vi "setUp.vi"(8 "error in (no error)":errorcluster, 11 "reference in":refnum<class "Configuration Tests.lvclass">) -> (0 "error out":errorcluster, 3 "reference out":refnum<class "Configuration Tests.lvclass">)   [LabVIEW 2017, in "Configuration Tests.lvclass"]
doc: "setUp runs prior to the test method during test execution. Use this method to initialize any object data required by your tests."
uses:
  Configuration Tests.lvclass
  C:/Program Files (x86)/National Instruments/LabVIEW 2017/vi.lib/addons/_JKI Toolkits/VI Tester/TestCase.llb/TestCase.lvclass
  Typedefs/DSF Engine Framework Configuration.ctl
  Typedefs/DSF Engine Plugin Configuration.ctl
  Typedefs/DSF Timing Info.ctl
  Typedefs/DSF Engine Plugin Thread Configuration.ctl
  Typedefs/DSF Settings Info.ctl
  Typedefs/DSF Engine Transfer Group Configuration.ctl
  Typedefs/DSF Direction.ctl
  Typedefs/DSF Engine Transfer Configuration.ctl
  Typedefs/DSF Byte Order.ctl
  Typedefs/DSF Engine Channel Configuration.ctl
  Typedefs/DSF Data Type.ctl
  Typedefs/DSF Timeout Behavior.ctl
  Configuration Tests.lvclass/Configuration Tests.ctl
  <vilib>/addons/_JKI Toolkits/VI Tester/TestCase.llb/TestCase.lvclass
  DSF Core.lvlib
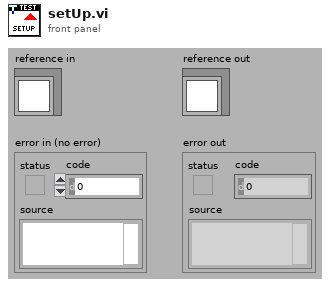
[diagram p1: front panel]
types:
  T1 = typedef "DSF Core.lvlib/DSF Engine Framework Configuration.ctl" = cluster{"plugins":T2[]}
  T2 = typedef "DSF Core.lvlib/DSF Engine Plugin Configuration.ctl" = cluster{"name":string, "components":string[], "cycle timing":T3, "threads":T4[], "transfer groups":T6[], "settings":T5}
  T3 = typedef "DSF Core.lvlib/DSF Timing Info.ctl" = cluster{"priority":u64, "decimation":u64, "offset":u64}
  T4 = typedef "DSF Core.lvlib/DSF Engine Plugin Thread Configuration.ctl" = cluster{"processor":i32, "priority offset":i16, "settings":T5}
  T5 = typedef "DSF Core.lvlib/DSF Settings Info.ctl" = cluster{"component":string, "name":string, "values":cluster{"key":string, "value":string}[]}[]
  T6 = typedef "DSF Core.lvlib/DSF Engine Transfer Group Configuration.ctl" = cluster{"name":string, "direction":T7, "cycle timing":T3, "thread index":u8, "settings":T5, "transfers":T8[], "timeout behavior":T12, "convert buffers":bool}
  T7 = typedef "DSF Core.lvlib/DSF Direction.ctl" = enum8{"Tx", "Rx"}
  T8 = typedef "DSF Core.lvlib/DSF Engine Transfer Configuration.ctl" = cluster{"name":string, "string byte order":T9, "settings":T5, "channels":T10[]}
  T9 = typedef "DSF Core.lvlib/DSF Byte Order.ctl" = enum8{"big-endian", "little-endian"}
  T10 = typedef "DSF Core.lvlib/DSF Engine Channel Configuration.ctl" = cluster{"string offset":u64, "name":string, "units":string, "engine data type":T11, "string data type":T11, "settings":T5}
  T11 = typedef "DSF Core.lvlib/DSF Data Type.ctl" = enum8{"Bool", "SGL", "DBL", "I8", "I16", "I32", "I64", "U8", "U16", "U32", "U64"}
  T12 = typedef "DSF Core.lvlib/DSF Timeout Behavior.ctl" = enum8{"Increment Late Count", "Throw Error"}
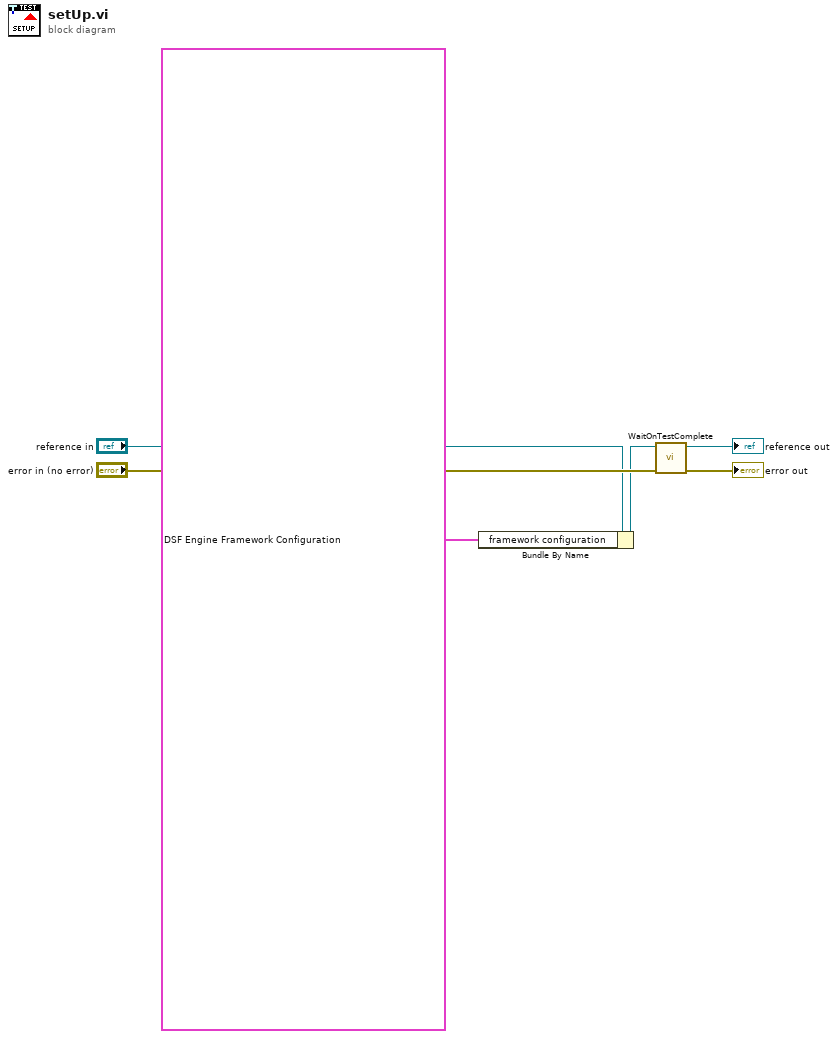
[diagram p0: block diagram]
diagram:
  n1 = Bundle By Name(cluster="reference in", "framework configuration"=T1 {"plugins"=[{"name"="Plugin", "components"=[], "cycle timing"={"priority"=10000, "decimation"=1, "offset"=0}, "threads"=[{"processor"=-2, "priority offset"=0, "settings"=[{"component"="a", "name"="a", "values"=[{"key"="a", "value"="a"}]}]}], "transfer groups"=[{"name"="Group", "direction"=enum."Tx", "cycle timing"={"priority"=100, "decimation"=1, "offset"=0}, "thread index"=255, "settings"=[{"component"="a", "name"="a", "values"=[{"key"="a", "value"="a"}]}], "transfers"=[{"name"="Transfer", "string byte order"=enum."big-endian", "settings"=[{"component"="a", "name"="a", "values"=[{"key"="a", "value"="a"}]}], "channels"=[{"string offset"=0, "name"="Channel", "units"="V", "engine data type"=enum."DBL", "string data type"=enum."DBL", "settings"=[]}, {"string offset"=0, "name"="Channel", "units"="V", "engine data type"=enum."DBL", "string data type"=enum."DBL", "settings"=[]}, {"string offset"=0, "name"="Channel", "units"="V", "engine data type"=enum."DBL", "string data type"=enum."DBL", "settings"=[]}, {"string offset"=0, "name"="Channel", "units"="V", "engine data type"=enum."DBL", "string data type"=enum."DBL", "settings"=[]}, {"string offset"=0, "name"="Channel", "units"="V", "engine data type"=enum."DBL", "string data type"=enum."DBL", "settings"=[]}, {"string offset"=0, "name"="Channel", "units"="V", "engine data type"=enum."DBL", "string data type"=enum."DBL", "settings"=[]}, {"string offset"=0, "name"="Channel", "units"="V", "engine data type"=enum."DBL", "string data type"=enum."DBL", "settings"=[]}, {"string offset"=0, "name"="Channel", "units"="V", "engine data type"=enum."DBL", "string data type"=enum."DBL", "settings"=[]}, {"string offset"=0, "name"="Channel", "units"="V", "engine data type"=enum."DBL", "string data type"=enum."DBL", "settings"=[]}, {"string offset"=0, "name"="Channel", "units"="V", "engine data type"=enum."DBL", "string data type"=enum."DBL", "settings"=[]}, {"string offset"=0, "name"="Channel", "units"="V", "engine data type"=enum."DBL", "string data type"=enum."DBL", "settings"=[]}, {"string offset"=0, "name"="Channel", "units"="V", "engine data type"=enum."DBL", "string data type"=enum."DBL", "settings"=[]}, {"string offset"=0, "name"="Channel", "units"="V", "engine data type"=enum."DBL", "string data type"=enum."DBL", "settings"=[]}, {"string offset"=0, "name"="Channel", "units"="V", "engine data type"=enum."DBL", "string data type"=enum."DBL", "settings"=[]}, {"string offset"=0, "name"="Channel", "units"="V", "engine data type"=enum."DBL", "string data type"=enum."DBL", "settings"=[]}, {"string offset"=0, "name"="Channel", "units"="V", "engine data type"=enum."DBL", "string data type"=enum."DBL", "settings"=[]}, {"string offset"=0, "name"="Channel", "units"="V", "engine data type"=enum."DBL", "string data type"=enum."DBL", "settings"=[]}, {"string offset"=0, "name"="Channel", "units"="V", "engine data type"=enum."DBL", "string data type"=enum."DBL", "settings"=[]}, {"string offset"=0, "name"="Channel", "units"="V", "engine data type"=enum."DBL", "string data type"=enum."DBL", "settings"=[]}, {"string offset"=0, "name"="Channel", "units"="V", "engine data type"=enum."DBL", "string data type"=enum."DBL", "settings"=[]}, {"string offset"=0, "name"="Channel", "units"="V", "engine data type"=enum."DBL", "string data type"=enum."DBL", "settings"=[]}, {"string offset"=0, "name"="Channel", "units"="V", "engine data type"=enum."DBL", "string data type"=enum."DBL", "settings"=[]}, {"string offset"=0, "name"="Channel", "units"="V", "engine data type"=enum."DBL", "string data type"=enum."DBL", "settings"=[]}, {"string offset"=0, "name"="Channel", "units"="V", "engine data type"=enum."DBL", "string data type"=enum."DBL", "settings"=[]}, {"string offset"=0, "name"="Channel", "units"="V", "engine data type"=enum."DBL", "string data type"=enum."DBL", "settings"=[]}, {"string offset"=0, "name"="Channel", "units"="V", "engine data type"=enum."DBL", "string data type"=enum."DBL", "settings"=[]}, {"string offset"=0, "name"="Channel", "units"="V", "engine data type"=enum."DBL", "string data type"=enum."DBL", "settings"=[]}, {"string offset"=0, "name"="Channel", "units"="V", "engine data type"=enum."DBL", "string data type"=enum."DBL", "settings"=[]}, {"string offset"=0, "name"="Channel", "units"="V", "engine data type"=enum."DBL", "string data type"=enum."DBL", "settings"=[]}, {"string offset"=0, "name"="Channel", "units"="V", "engine data type"=enum."DBL", "string data type"=enum."DBL", "settings"=[]}, {"string offset"=0, "name"="Channel", "units"="V", "engine data type"=enum."DBL", "string data type"=enum."DBL", "settings"=[]}, {"string offset"=0, "name"="Channel", "units"="V", "engine data type"=enum."DBL", "string data type"=enum."DBL", "settings"=[]}, {"string offset"=0, "name"="Channel", "units"="V", "engine data type"=enum."DBL", "string data type"=enum."DBL", "settings"=[]}, {"string offset"=0, "name"="Channel", "units"="V", "engine data type"=enum."DBL", "string data type"=enum."DBL", "settings"=[]}, {"string offset"=0, "name"="Channel", "units"="V", "engine data type"=enum."DBL", "string data type"=enum."DBL", "settings"=[]}, {"string offset"=0, "name"="Channel", "units"="V", "engine data type"=enum."DBL", "string data type"=enum."DBL", "settings"=[]}, {"string offset"=0, "name"="Channel", "units"="V", "engine data type"=enum."DBL", "string data type"=enum."DBL", "settings"=[]}, {"string offset"=0, "name"="Channel", "units"="V", "engine data type"=enum."DBL", "string data type"=enum."DBL", "settings"=[]}, {"string offset"=0, "name"="Channel", "units"="V", "engine data type"=enum."DBL", "string data type"=enum."DBL", "settings"=[]}, {"string offset"=0, "name"="Channel", "units"="V", "engine data type"=enum."DBL", "string data type"=enum."DBL", "settings"=[]}, {"string offset"=0, "name"="Channel", "units"="V", "engine data type"=enum."DBL", "string data type"=enum."DBL", "settings"=[]}, {"string offset"=0, "name"="Channel", "units"="V", "engine data type"=enum."DBL", "string data type"=enum."DBL", "settings"=[]}, {"string offset"=0, "name"="Channel", "units"="V", "engine data type"=enum."DBL", "string data type"=enum."DBL", "settings"=[]}, {"string offset"=0, "name"="Channel", "units"="V", "engine data type"=enum."DBL", "string data type"=enum."DBL", "settings"=[]}, {"string offset"=0, "name"="Channel", "units"="V", "engine data type"=enum."DBL", "string data type"=enum."DBL", "settings"=[]}, {"string offset"=0, "name"="Channel", "units"="V", "engine data type"=enum."DBL", "string data type"=enum."DBL", "settings"=[]}, {"string offset"=0, "name"="Channel", "units"="V", "engine data type"=enum."DBL", "string data type"=enum."DBL", "settings"=[]}, {"string offset"=0, "name"="Channel", "units"="V", "engine data type"=enum."DBL", "string data type"=enum."DBL", "settings"=[]}, {"string offset"=0, "name"="Channel", "units"="V", "engine data type"=enum."DBL", "string data type"=enum."DBL", "settings"=[]}, {"string offset"=0, "name"="Channel", "units"="V", "engine data type"=enum."DBL", "string data type"=enum."DBL", "settings"=[]}, {"string offset"=0, "name"="Channel", "units"="V", "engine data type"=enum."DBL", "string data type"=enum."DBL", "settings"=[]}, {"string offset"=0, "name"="Channel", "units"="V", "engine data type"=enum."DBL", "string data type"=enum."DBL", "settings"=[]}, {"string offset"=0, "name"="Channel", "units"="V", "engine data type"=enum."DBL", "string data type"=enum."DBL", "settings"=[]}, {"string offset"=0, "name"="Channel", "units"="V", "engine data type"=enum."DBL", "string data type"=enum."DBL", "settings"=[]}, {"string offset"=0, "name"="Channel", "units"="V", "engine data type"=enum."DBL", "string data type"=enum."DBL", "settings"=[]}, {"string offset"=0, "name"="Channel", "units"="V", "engine data type"=enum."DBL", "string data type"=enum."DBL", "settings"=[]}, {"string offset"=0, "name"="Channel", "units"="V", "engine data type"=enum."DBL", "string data type"=enum."DBL", "settings"=[]}, {"string offset"=0, "name"="Channel", "units"="V", "engine data type"=enum."DBL", "string data type"=enum."DBL", "settings"=[]}, {"string offset"=0, "name"="Channel", "units"="V", "engine data type"=enum."DBL", "string data type"=enum."DBL", "settings"=[]}, {"string offset"=0, "name"="Channel", "units"="V", "engine data type"=enum."DBL", "string data type"=enum."DBL", "settings"=[]}, {"string offset"=0, "name"="Channel", "units"="V", "engine data type"=enum."DBL", "string data type"=enum."DBL", "settings"=[]}, {"string offset"=0, "name"="Channel", "units"="V", "engine data type"=enum."DBL", "string data type"=enum."DBL", "settings"=[]}, {"string offset"=0, "name"="Channel", "units"="V", "engine data type"=enum."DBL", "string data type"=enum."DBL", "settings"=[]}, {"string offset"=0, "name"="Channel", "units"="V", "engine data type"=enum."DBL", "string data type"=enum."DBL", "settings"=[]}, {"string offset"=0, "name"="Channel", "units"="V", "engine data type"=enum."DBL", "string data type"=enum."DBL", "settings"=[]}, {"string offset"=0, "name"="Channel", "units"="V", "engine data type"=enum."DBL", "string data type"=enum."DBL", "settings"=[]}, {"string offset"=0, "name"="Channel", "units"="V", "engine data type"=enum."DBL", "string data type"=enum."DBL", "settings"=[]}, {"string offset"=0, "name"="Channel", "units"="V", "engine data type"=enum."DBL", "string data type"=enum."DBL", "settings"=[]}, {"string offset"=0, "name"="Channel", "units"="V", "engine data type"=enum."DBL", "string data type"=enum."DBL", "settings"=[]}, {"string offset"=0, "name"="Channel", "units"="V", "engine data type"=enum."DBL", "string data type"=enum."DBL", "settings"=[]}, {"string offset"=0, "name"="Channel", "units"="V", "engine data type"=enum."DBL", "string data type"=enum."DBL", "settings"=[]}, {"string offset"=0, "name"="Channel", "units"="V", "engine data type"=enum."DBL", "string data type"=enum."DBL", "settings"=[]}, {"string offset"=0, "name"="Channel", "units"="V", "engine data type"=enum."DBL", "string data type"=enum."DBL", "settings"=[]}, {"string offset"=0, "name"="Channel", "units"="V", "engine data type"=enum."DBL", "string data type"=enum."DBL", "settings"=[]}, {"string offset"=0, "name"="Channel", "units"="V", "engine data type"=enum."DBL", "string data type"=enum."DBL", "settings"=[]}, {"string offset"=0, "name"="Channel", "units"="V", "engine data type"=enum."DBL", "string data type"=enum."DBL", "settings"=[]}, {"string offset"=0, "name"="Channel", "units"="V", "engine data type"=enum."DBL", "string data type"=enum."DBL", "settings"=[]}, {"string offset"=0, "name"="Channel", "units"="V", "engine data type"=enum."DBL", "string data type"=enum."DBL", "settings"=[]}, {"string offset"=0, "name"="Channel", "units"="V", "engine data type"=enum."DBL", "string data type"=enum."DBL", "settings"=[]}, {"string offset"=0, "name"="Channel", "units"="V", "engine data type"=enum."DBL", "string data type"=enum."DBL", "settings"=[]}, {"string offset"=0, "name"="Channel", "units"="V", "engine data type"=enum."DBL", "string data type"=enum."DBL", "settings"=[]}, {"string offset"=0, "name"="Channel", "units"="V", "engine data type"=enum."DBL", "string data type"=enum."DBL", "settings"=[]}, {"string offset"=0, "name"="Channel", "units"="V", "engine data type"=enum."DBL", "string data type"=enum."DBL", "settings"=[]}, {"string offset"=0, "name"="Channel", "units"="V", "engine data type"=enum."DBL", "string data type"=enum."DBL", "settings"=[]}, {"string offset"=0, "name"="Channel", "units"="V", "engine data type"=enum."DBL", "string data type"=enum."DBL", "settings"=[]}, {"string offset"=0, "name"="Channel", "units"="V", "engine data type"=enum."DBL", "string data type"=enum."DBL", "settings"=[]}, {"string offset"=0, "name"="Channel", "units"="V", "engine data type"=enum."DBL", "string data type"=enum."DBL", "settings"=[]}, {"string offset"=0, "name"="Channel", "units"="V", "engine data type"=enum."DBL", "string data type"=enum."DBL", "settings"=[]}, {"string offset"=0, "name"="Channel", "units"="V", "engine data type"=enum."DBL", "string data type"=enum."DBL", "settings"=[]}, {"string offset"=0, "name"="Channel", "units"="V", "engine data type"=enum."DBL", "string data type"=enum."DBL", "settings"=[]}, {"string offset"=0, "name"="Channel", "units"="V", "engine data type"=enum."DBL", "string data type"=enum."DBL", "settings"=[]}, {"string offset"=0, "name"="Channel", "units"="V", "engine data type"=enum."DBL", "string data type"=enum."DBL", "settings"=[]}, {"string offset"=0, "name"="Channel", "units"="V", "engine data type"=enum."DBL", "string data type"=enum."DBL", "settings"=[]}, {"string offset"=0, "name"="Channel", "units"="V", "engine data type"=enum."DBL", "string data type"=enum."DBL", "settings"=[]}, {"string offset"=0, "name"="Channel", "units"="V", "engine data type"=enum."DBL", "string data type"=enum."DBL", "settings"=[]}, {"string offset"=0, "name"="Channel", "units"="V", "engine data type"=enum."DBL", "string data type"=enum."DBL", "settings"=[]}, {"string offset"=0, "name"="Channel", "units"="V", "engine data type"=enum."DBL", "string data type"=enum."DBL", "settings"=[]}, {"string offset"=0, "name"="Channel", "units"="V", "engine data type"=enum."DBL", "string data type"=enum."DBL", "settings"=[]}, {"string offset"=0, "name"="Channel", "units"="V", "engine data type"=enum."DBL", "string data type"=enum."DBL", "settings"=[]}, {"string offset"=0, "name"="Channel", "units"="V", "engine data type"=enum."DBL", "string data type"=enum."DBL", "settings"=[{"component"="a", "name"="a", "values"=[{"key"="a", "value"="a"}]}]}]}], "timeout behavior"=enum."Increment Late Count", "convert buffers"=TRUE}], "settings"=[{"component"="a", "name"="a", "values"=[{"key"="a", "value"="a"}]}]}]}) -> (w2:refnum<class "Configuration Tests.lvclass">)
  n2 = call <vilib>:"WaitOnTestComplete.vi"("error in (no error)"="error in (no error)", "TestCase in"=w2) -> ("error out"=→"error out":errorcluster, "TestCase out"=→"reference out":refnum<class "Configuration Tests.lvclass">)  [unwired: 8 in]
